vi "Error handler.vi"(3 "Recieved Packet":string) -> (0 "Ошибка?":bool, 1 "Error":string)   [LabVIEW 2017, in "LV_Unicorn.lvlib"]
uses:
  LV_Unicorn.lvlib
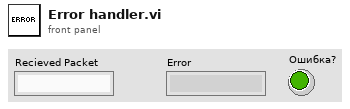
[diagram p1: front panel]
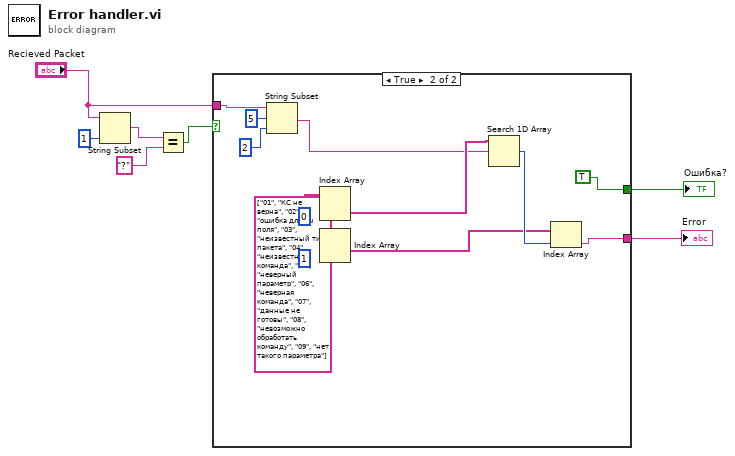
[diagram p0: block diagram]
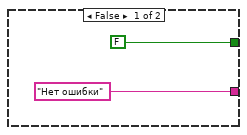
[diagram p2: hidden frame]
diagram:
  n1 = String Subset(string="Recieved Packet", length (rest)=1 ("length (rest)")) -> (substring=w4:string)  [unwired: 1 in]
  n2 = Equal?(x=w4, y="?") -> (x = y?=w2:bool)
  n3 = case shown="True" w2 {
    tunnel: "Recieved Packet" -> [_ w21]
    tunnel: ["Нет ошибки" w11] -> w6
    tunnel: [FALSE TRUE] -> w1
    frame False {
    }
    frame True {
      w18 = string[][] [["01", "КС не верна"], ["02", "ошибка длины поля"], ["03", "неизвестный тип пакета"], ["04", "неизвестная команда"], ["05", "неверный параметр"], ["06", "неверная команда"], ["07", "данные не готовы"], ["08", "невозможно обработать команду"], ["09", "нет такого параметра"]]
      n4 = String Subset(string=w21, offset (0)=5, length (rest)=2 ("length (rest)")) -> (substring=w14:string)
      n5 = Index Array(array=w18, index (col)=0 ("disabled index (col)")) -> (element=w15:string[])  [unwired: 1 in]
      n6 = Index Array(array=w18, index (col)=1 ("disabled index (col)")) -> (element=w12:string[])  [unwired: 1 in]
      n7 = Search 1D Array(1D array=w15, element=w14) -> (index of element=w13:i32)  [unwired: 1 in]
      n8 = Index Array(array=w12, index=w13) -> (element=w11:string)
    }
  }
  "Error" <- w6
  "Ошибка?" <- w1
